vi "noise_cancellation.vi"() -> ()   [LabVIEW 2020]
uses:
  <vilib>/ptbypt/NI_PtbyPt.lvlib
panel:
  out "LSE1,LSE2":cluster{dbl, dbl}(graph)
  in  "standard deviation":dbl=1.0 format="%0.2f"
  out "LMS Filter 2":dbl[](array[numeric])
  out "LMS Filter 1":dbl[](array[numeric])
  out "Error e[n] 2":dbl(graph)
  out "Error e[n] 1":dbl(graph)
  in  "Adaptive Filter Length":i32
  in  "milliseconds to wait":u32
  in  "FIR Filter Coefficients":dbl[](array[numeric])
  in  "stop":bool
  in  "LMS Filter2 Step Size, mu":dbl
  in  "LMS Filter1 Step Size, mu":dbl
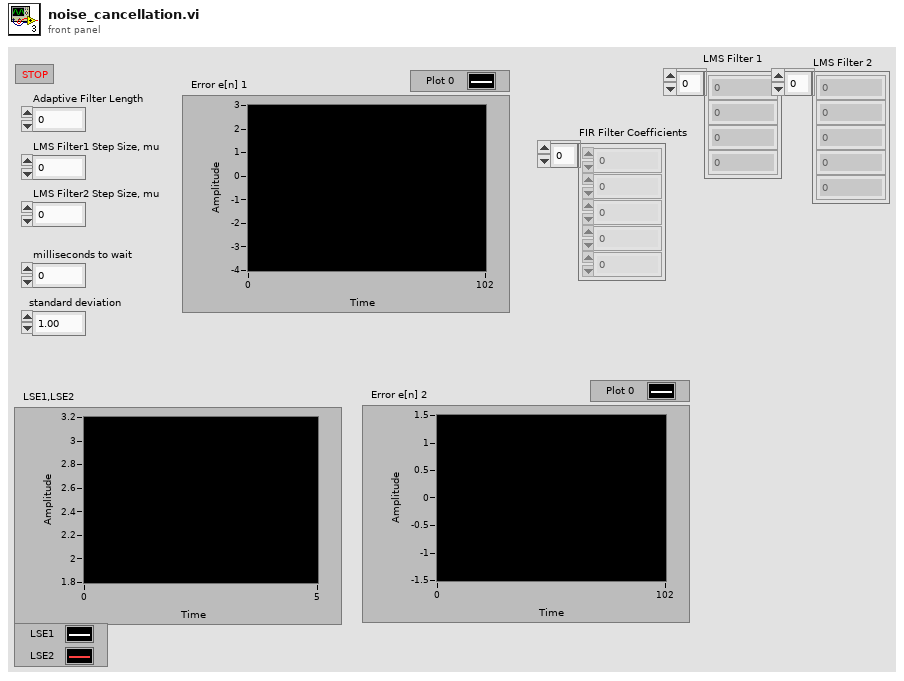
[diagram p1: front panel]
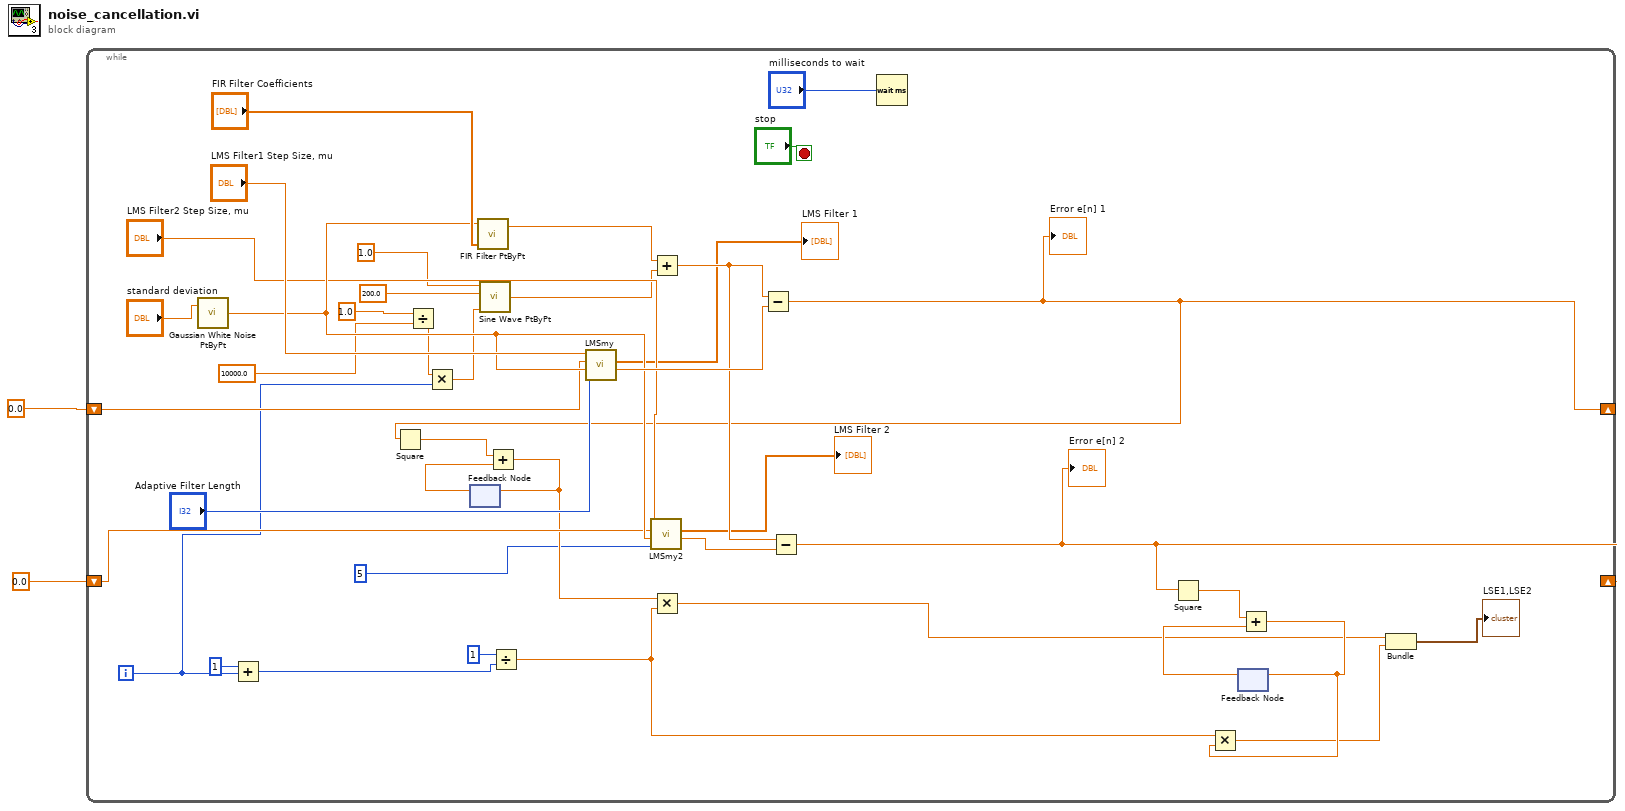
[diagram p0: block diagram]
diagram:
  n1 = while {
    shift-right: [w20] -> _
    shift-left: 0.0 -> [w24]
    shift-right: [w27] -> _
    shift-left: 0.0 -> [w35]
    i -> [w5]
    stop <- "stop" stop-if-true
    n2 = call <vilib>:"Gaussian White Noise PtByPt.vi"("standard deviation"="standard deviation") -> ("Gaussian white noise"=w36:dbl)  [unwired: 2 in]
    n3 = Add(x=1, y=w5) -> (x+y=w25:i32)
    n4 = Divide(x=1.0, y=10000.0) -> (x/y=w4:dbl)
    n5 = Multiply(x=w4, y=w5) -> (x*y=w3:dbl)
    n6 = feedback #1() -> (w22:dbl)  [unwired: 1 in]
    n7 = call <vilib>:"FIR Filter PtByPt.vi"("Forward Coefficients"="FIR Filter Coefficients", "x"=w36) -> ("Filtered x"=w39:dbl)  [unwired: 2 in, 1 out]
    n8 = call <vilib>:"Sine Wave PtByPt.vi"("time"=w3, "frequency"=200.0, "amplitude"=1.0) -> ("sine wave"=w10:dbl)  [unwired: 1 in]
    n9 = Divide(x=1, y=w25) -> (x/y=w17:dbl)
    n10 = call "LMSmy.vi"("sample length"="Adaptive Filter Length", "x(n+1) input point"=w36, "error e(n)"=w24, "mu"="LMS Filter1 Step Size, mu") -> ("y(n+1)"=w38:dbl, "w(n)"=→"LMS Filter 1":dbl[])  [unwired: 6 in]
    n11 = call "LMSmy2.vi"("sample length"=5, "x(n+1) input point"=w36, "error e(n)"=w35, "mu"="LMS Filter2 Step Size, mu") -> ("y(n+1)"=w33:dbl, "w(n)"=→"LMS Filter 2":dbl[])  [unwired: 6 in]
    n12 = Add(x=w39, y=w10) -> (x+y=w34:dbl)
    n13 = Subtract(x=w34, y=w38) -> (x-y=w20:dbl)
    "Error e[n] 1" <- w20
    n14 = Square(x=w20) -> (x^2=w23:dbl)
    n15 = Add(x=w23, y=w22) -> (x+y=w21:dbl)
    n16 = feedback-in #1(w21) -> ()
    n17 = Multiply(x=w21, y=w17) -> (x*y=w15:dbl)
    n18 = Subtract(x=w34, y=w33) -> (x-y=w27:dbl)
    "Error e[n] 2" <- w27
    n19 = Wait (ms)(milliseconds to wait="milliseconds to wait") -> ()  [unwired: 1 out]
    n20 = Square(x=w27) -> (x^2=w19:dbl)
    n21 = feedback #2() -> (w18:dbl)  [unwired: 1 in]
    n22 = Add(x=w19, y=w18) -> (x+y=w16:dbl)
    n23 = Multiply(x=w17, y=w16) -> (x*y=w14:dbl)
    n24 = feedback-in #2(w16) -> ()
    n25 = Bundle(w15, w14) -> (→"LSE1,LSE2":cluster{dbl, dbl})  [unwired: 1 in]
  }
